vi "SQL_Login_Maintenance.vi"(9 "UsersTable":string, 11 "ConnectionDSN":string) -> (1 "qLevel":i32, 3 "User":string)   [LabVIEW 2017]
uses:
  <vilib>/event_ctls.llb/eventvkey.ctl
panel:
  out "Role":string
  out "Department":string
  out "Level":string
  in  "Cancel Button":bool
  in  "OK Button":bool
  in  "Password":string
  in  "UserName":u16(ring) items=["BenitoSanchez", "Edgar", "IvanReyes", "Quality", "SalvadorGonzalez", "Sergio"]
  # "Plase, fill your data to login"
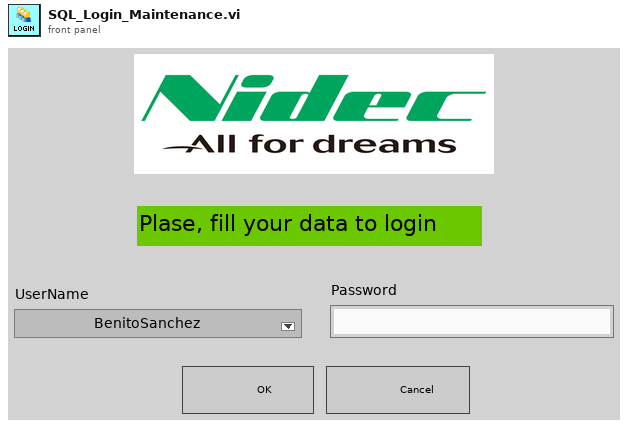
[diagram p1: front panel]
types:
  T1 = typedef "eventvkey.ctl" = enum16{"ASCII", "Enter", "Return", "Shift", "Ctrl", "Alt", "Cmd", "Opt", "Caps", "NumLock", "Clear", "Break", "Up", "Down", "Left", "Right", "Insert", "Delete", "Home", "End", "PageUp", "PageDown", "Escape", "Help", "Pause", "ScrollLock", "F1", "F2", "F3", "F4", "F5", "F6", "F7", "F8", "F9", "F10", "F11", "F12", "F13", "F14", "F15", "F16", "F17", "F18", "F19", "F20", "F21", "F22", "F23", "F24", "Play", "VolumeUp", "VolumeDown", "Mute", "Two Byte Char"}
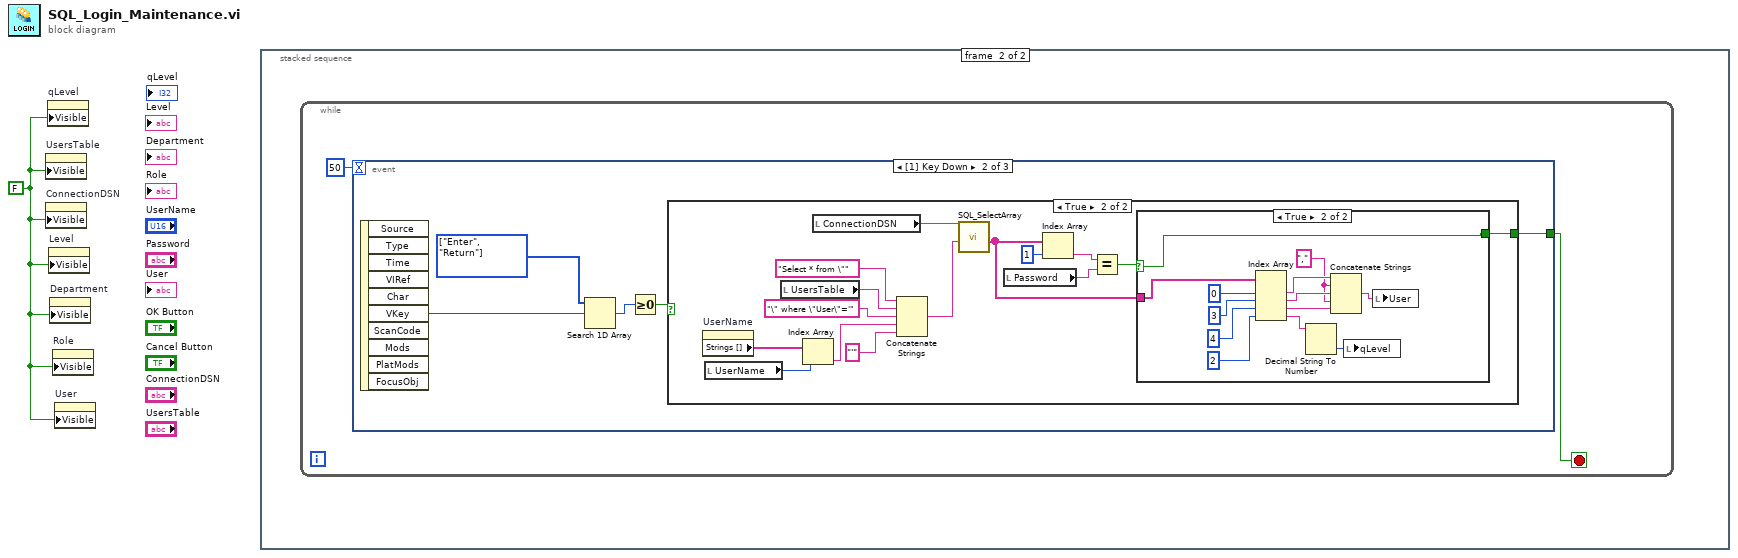
[diagram p0: block diagram]
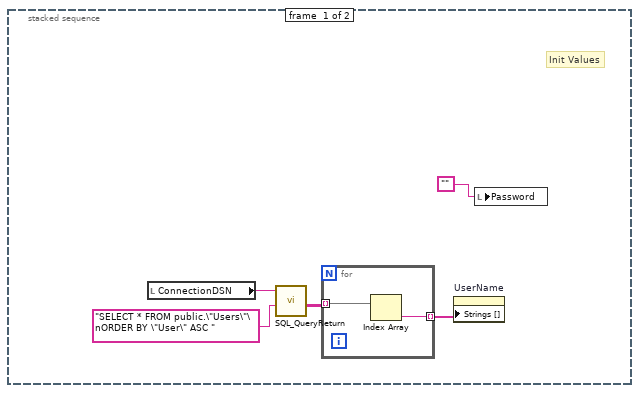
[diagram p2: hidden frame]
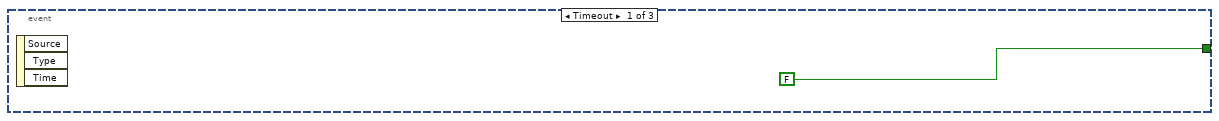
[diagram p3: hidden frame]
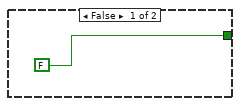
[diagram p4: hidden frame]
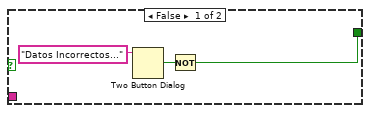
[diagram p5: hidden frame]
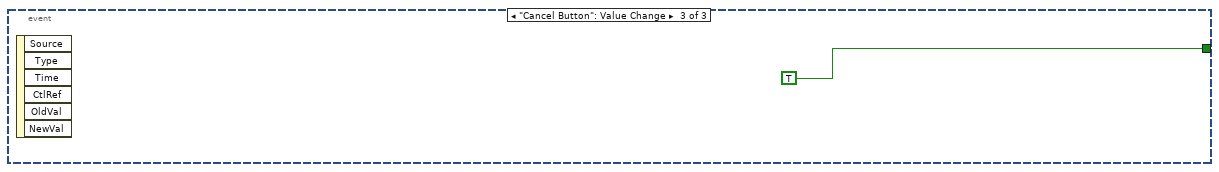
[diagram p6: hidden frame]
diagram:
  w1 = FALSE
  n1 = property on="UsersTable" class="Str"("Visible"=w1) -> ()  [unwired: 2 in, 2 out]
  n2 = property on="ConnectionDSN" class="Str"("Visible"=w1) -> ()  [unwired: 2 in, 2 out]
  n3 = property on="qLevel" class="DigNum (strict)"("Visible"=w1) -> ()  [unwired: 2 in, 2 out]
  n4 = property on="Level" class="Str"("Visible"=w1) -> ()  [unwired: 2 in, 2 out]
  n5 = property on="Department" class="Str"("Visible"=w1) -> ()  [unwired: 2 in, 2 out]
  n6 = property on="Role" class="Str"("Visible"=w1) -> ()  [unwired: 2 in, 2 out]
  n7 = property on="User" class="Str"("Visible"=w1) -> ()  [unwired: 2 in, 2 out]
  n8 = stacked-sequence {
    frame #0 {
      # "Init Values"
      n9 = local read "ConnectionDSN"() -> (w4:string)
      n10 = call "SQL_QueryReturn.vi"("SQL query"="SELECT * FROM public.\"Users\"\nORDER BY \"User\" ASC ", "ConnectionDSN"=w4) -> ("data"=w5:string[][])  [unwired: 9 in]
      n11 = for {
        tunnel: w5 -> [w8] mode=indexing
        tunnel: [w7] -> w2 mode=indexing
        n12 = Index Array(array=w8) -> (element=w7:string)  [unwired: 1 in]
      }
      n13 = property on="UserName" class="Ring (strict)"("Strings []"=w2) -> ()  [unwired: 2 in, 2 out]
      n14 = local write "Password"("") -> ()
    }
    frame #1 {
      n15 = while {
        stop <- w9 stop-if-true
        n16 = event shown="[1] Key Down" {
          selector: _ -> [_ _ _]
          dyn-events: _ -> [_ _ _]
          timeout: 50 -> [_ _ _]
          tunnel: [FALSE w16 TRUE] -> w9
          event Timeout {
            n17 = event-data() -> ()  [unwired: 1 in, 3 out]
          }
          event Key Down {
            w14 = T1[] [enum."Enter", enum."Return"] items=["ASCII", "Enter", "Return", "Shift", "Ctrl", "Alt", "Cmd", "Opt", "Caps", "NumLock", "Clear", "Break", "Up", "Down", "Left", "Right", "Insert", "Delete", "Home", "End", "PageUp", "PageDown", "Escape", "Help", "Pause", "ScrollLock", "F1", "F2", "F3", "F4", "F5", "F6", "F7", "F8", "F9", "F10", "F11", "F12", "F13", "F14", "F15", "F16", "F17", "F18", "F19", "F20", "F21", "F22", "F23", "F24", "Play", "VolumeUp", "VolumeDown", "Mute", "Two Byte Char"]
            n18 = event-data() -> ("VKey"=w15:T1)  [unwired: 1 in, 9 out]
            n19 = Search 1D Array(1D array=w14, element=w15) -> (index of element=w13:i32)  [unwired: 1 in]
            n20 = Greater Or Equal To 0?(x=w13) -> (x >= 0?=w12:bool)
            n21 = case shown="True" w12 {
              tunnel: [FALSE w22] -> w16
              frame False {
              }
              frame True {
                n22 = property on="UserName" class="Ring (strict)"() -> ("Strings []"=w20:string[])  [unwired: 2 in, 2 out]
                n23 = local read "UserName"() -> (w19:u16)
                n24 = local read "UsersTable"() -> (w30:string)
                n25 = Index Array(array=w20, index=w19) -> (element=w18:string)
                n26 = local read "ConnectionDSN"() -> (w32:string)
                n27 = Concatenate Strings("Select * from \"", w30, "\" where \"User\"='", w18, "'") -> (w27:string)
                n28 = call "SQL_SelectArray.vi"("SQL query"=w27, "ConnectionDSN"=w32) -> ("data"=w21:string[])  [unwired: 9 in]
                n29 = local read "Password"() -> (w25:string)
                n30 = Index Array(array=w21, index=1) -> (element=w24:string)
                n31 = Equal?(x=w24, y=w25) -> (x = y?=w23:bool)
                n32 = case shown="True" w23 {
                  selector: w23 -> [_ w48]
                  tunnel: [w34 w48] -> w22
                  tunnel: w21 -> [_ w47]
                  frame False {
                    n33 = Two Button Dialog(message="Datos Incorrectos...") -> (T button?=w33:bool)  [unwired: 2 in]
                    n34 = Not(x=w33) -> (.not. x?=w34:bool)
                  }
                  frame True {
                    w41 = ","
                    n35 = Index Array(array=w47, index #1=0, index #2=3, index #3=4, index #4=2) -> (element #1=w43:string, element #2=w42:string, element #3=w40:string, element #4=w37:string)
                    n36 = Decimal String To Number(string=w37) -> (number=w36:i32)  [unwired: 2 in, 1 out]
                    n37 = Concatenate Strings(w43, w41, w42, w41, w40) -> (w39:string)
                    n38 = local write "qLevel"(w36) -> ()
                    n39 = local write "User"(w39) -> ()
                  }
                }
              }
            }
          }
          event "Cancel Button": Value Change {
            n40 = event-data() -> ()  [unwired: 1 in, 6 out]
          }
        }
      }
    }
  }
